vi "to string.vi"(8 "error in":errorcluster, 11 "configuration in":refnum<class "channel config object.lvclass">) -> (0 "error out":errorcluster, 1 "data":string, 2 "version":string, 3 "configuration out":refnum<class "channel config object.lvclass">)   [LabVIEW 2013, in "channel config object.lvclass"]
doc: "Provides an interface for saving a module configuration to a file or other serialized data source. It is recommended that all children of this class store data in two sets--data required for its own initialization, and any data required for parent initialization--and that each implementation uses the <b>Call Parent Method</b> primitive to serialize parent information."
uses:
  channel config object.lvclass
  CEF_TreeControl/serializable configuration/NISE_CEF_serializable configuration.lvclass
  channel config object.lvclass/channel config object.ctl
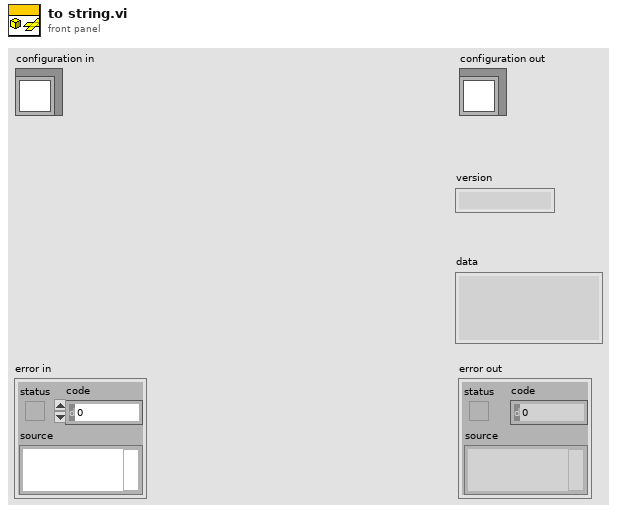
[diagram p1: front panel]
types:
  T1 = typedef "channel config object.lvclass/ChannelData.ctl" = cluster{"channel group":string, "channel name":string, "IO":string, "sensor ID":string, "description":string, "system":string, "channel type":string}
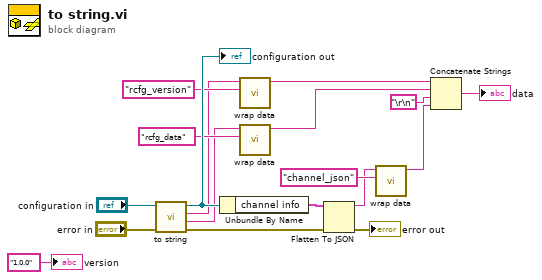
[diagram p0: block diagram]
diagram:
  n1 = call-parent "to string.vi"("error in"="error in", "configuration in"="configuration in") -> ("error out"=w11:errorcluster, "data"=w2:string, "version"=w1:string, "configuration out"=w15:refnum<class "channel config object.lvclass">)  [unwired: 6 in]
  "configuration out" <- w15
  n2 = Unbundle By Name(w15) -> ("channel info"=w12:T1)
  n3 = call "wrap data.vi"("identifier"="rcfg_version" ("additional identifier"), "data to wrap"=w1) -> ("wrapped data"=w7:string)  [unwired: 9 in]
  n4 = call "wrap data.vi"("identifier"="rcfg_data" ("additional identifier"), "data to wrap"=w2) -> ("wrapped data"=w6:string)  [unwired: 9 in]
  n5 = Flatten To JSON(anything=w12, error in (no error)=w11) -> (JSON string=w8:string, 11:→"error out":errorcluster)  [unwired: 1 in]
  n6 = call "wrap data.vi"("identifier"="channel_json" ("additional identifier"), "data to wrap"=w8) -> ("wrapped data"=w4:string)  [unwired: 9 in]
  n7 = Concatenate Strings(w7, w6, "\r\n", w4) -> (→"data":string)
  "version" <- "1.0.0" ("version")
